vi "Read Props.vi"(8 "error in (no error)":errorcluster, 11 "CheckboxControlEditorPanel in":refnum<class "CheckboxControlEditorPanel.lvclass">) -> (0 "error out":errorcluster, 2 "Props":T1, 3 "CheckboxControlEditorPanel out":refnum<class "CheckboxControlEditorPanel.lvclass">)   [LabVIEW 2020, in "VolatusGUIControls.lvlib" / "CheckboxControlEditorPanel.lvclass"]
uses:
  CheckboxControlEditorPanel.lvclass
  Props.ctl
  JSON Props.ctl
  VolatusGUIEditorCore/Label Props.ctl
  VolatusGUIEditorCore/Position Props.ctl
  VolatusGUIEditorCore/Boolean Color Props.ctl
  CheckboxControlEditorPanel.lvclass/CheckboxControlEditorPanel.ctl
  6192d86b-95f4-4395-a51d-5e2cf281f57a.vi
  <vilib>/JDP Science/JSONtext/JSON text to Variant.vi
  <vilib>/JDP Science/JSONtext/LVClass Serializer/JSONtext LVClass Serializer.lvclass
  VolatusGUIControls.lvlib
  VolatusGUIEditorCore/VolatusGUIEditorCore.lvlib
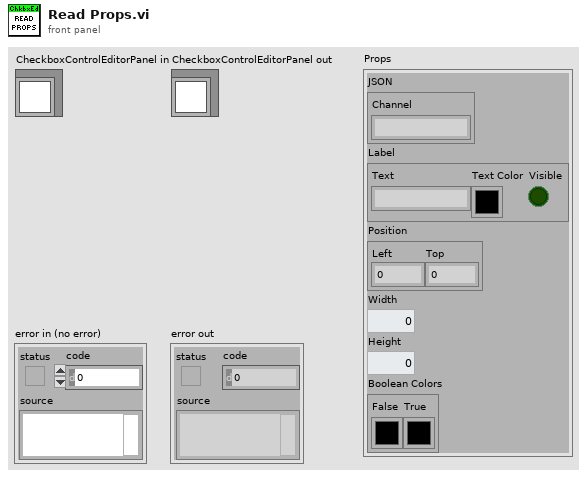
[diagram p1: front panel]
types:
  T1 = typedef "VolatusGUIControls.lvlib/CheckboxControlEditorPanel.lvclass/Props.ctl" = cluster{"JSON":T2, "Label":T3, "Position":T4, "Width":u16, "Height":u16, "Boolean Colors":T5}
  T2 = typedef "VolatusGUIControls.lvlib/CheckboxControlEditorPanel.lvclass/JSON Props.ctl" = cluster{"Channel":string}
  T3 = typedef "VolatusGUIEditorCore.lvlib/Label Props.ctl" = cluster{"Text":string, "Text Color":u32, "Visible":bool}
  T4 = typedef "VolatusGUIEditorCore.lvlib/Position Props.ctl" = cluster{"Left":i32, "Top":i32}
  T5 = typedef "VolatusGUIEditorCore.lvlib/Boolean Color Props.ctl" = cluster{"False":u32, "True":u32}
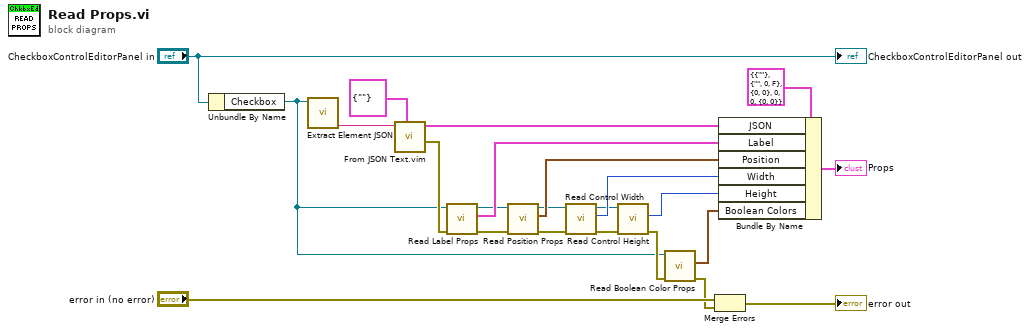
[diagram p0: block diagram]
diagram:
  n1 = Unbundle By Name("CheckboxControlEditorPanel in") -> ("Checkbox"=w4:refnum<vi>)
  n2 = call "Extract Element JSON.vi"("Ctl Refnum in"=w4) -> ("JSON"=w22:string)  [unwired: 7 in, 3 out]
  n3 = call "From JSON Text.vim"("Data Type and Default Value"=T2 {"Channel"=""} ("JSON Props"), "JSON"=w22) -> ("error out"=w16:errorcluster, "Data out"=w17:T2)  [unwired: 8 in]
  n4 = call "Read Label Props.vi"("error in (no error)"=w16, "Ctl Refnum in"=w4) -> ("error out"=w14:errorcluster, "Label Props"=w15:T3, "Ctl Refnum"=w13:refnum<vi>)  [unwired: 7 in]
  n5 = call "Read Position Props.vi"("error in (no error)"=w14, "Ctl Refnum in"=w13) -> ("error out"=w11:errorcluster, "Position Props"=w12:T4, "Ctl Refnum"=w10:refnum<vi>)  [unwired: 7 in]
  n6 = call "Read Control Width.vi"("error in"=w11, "Control in"=w10) -> ("error out"=w8:errorcluster, "Width"=w9:u32, "Control"=w7:refnum<vi>)  [unwired: 7 in]
  n7 = call "Read Control Height.vi"("error in"=w8, "Control in"=w7) -> ("error out"=w5:errorcluster, "Height"=w6:u32)  [unwired: 7 in, 1 out]
  n8 = call "Read Boolean Color Props.vi"("error in (no error)"=w5, "Control in"=w4) -> ("error out"=w1:errorcluster, "Boolean Colors Props"=w3:T5)  [unwired: 7 in, 1 out]
  n9 = Merge Errors("error in (no error)", w1) -> (→"error out":errorcluster)
  n10 = Bundle By Name(cluster=T1 {"JSON"={"Channel"=""}, "Label"={"Text"="", "Text Color"=0, "Visible"=FALSE}, "Position"={"Left"=0, "Top"=0}, "Width"=0, "Height"=0, "Boolean Colors"={"False"=0, "True"=0}} ("Props"), "JSON"=w17, "Label"=w15, "Position"=w12, "Width"=w9, "Height"=w6, "Boolean Colors"=w3) -> (→"Props":T1)
  "CheckboxControlEditorPanel out" <- "CheckboxControlEditorPanel in"
